vi "mono_camera.vi"(8 "error in":errorcluster, 11 "tcp_in":refnum<k5>) -> (0 "error out":errorcluster, 2 "camera_out":picture, 3 "tcp_out":refnum<k5>)   [LabVIEW 2018]
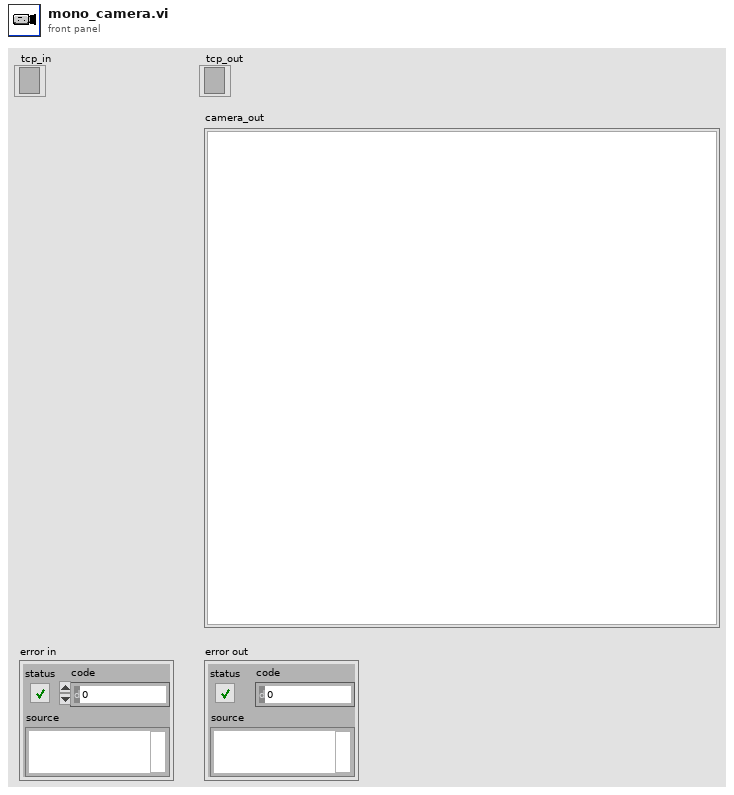
[diagram p1: front panel]
types:
  T1 = typedef "imagedata.ctl" = cluster{"image type":i32, "image depth":i32, "image":u8[], "mask":u8[], "colors":u32[], "Rectangle":cluster{"left":i16, "top":i16, "right":i16, "bottom":i16}}
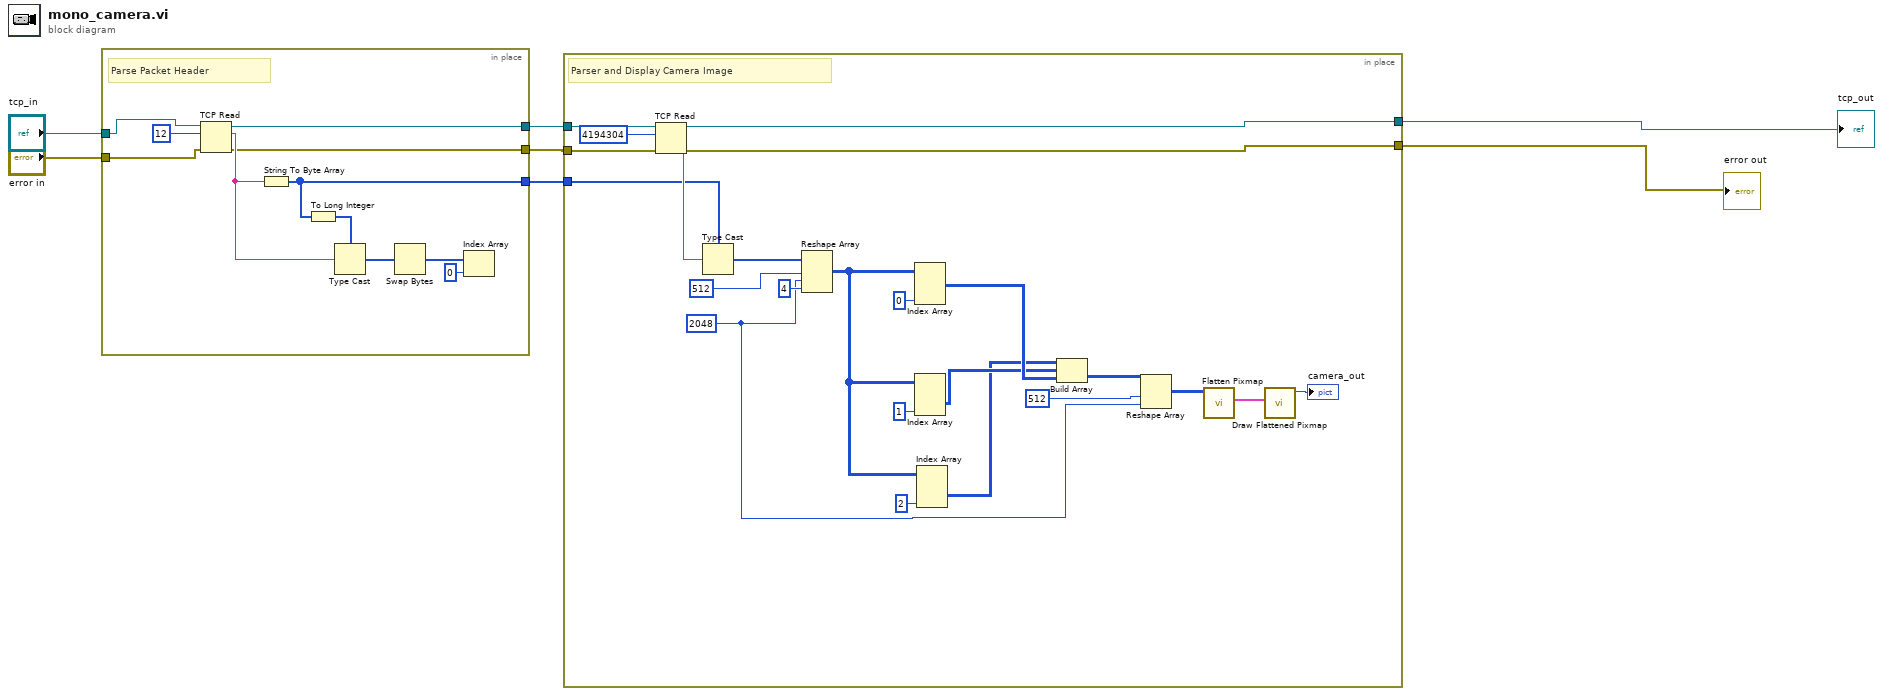
[diagram p0: block diagram]
diagram:
  n1 = in-place "Parse Header" {
    in-place-border: [w15] -> w1
    in-place-border: [w14] -> w2
    in-place-border: [w12] -> w3
    in-place-border: "error in" -> [w11]
    in-place-border: "tcp_in" -> [w10]
    # "Parse Packet Header"
    n2 = TCP Read(connection ID=w10, bytes to read=12, error in (no error)=w11) -> (connection ID out=w15:refnum<k5>, data out=w17:string, error out=w14:errorcluster)  [unwired: 2 in]
    n3 = String To Byte Array(string=w17) -> (unsigned byte array=w12:u8[])
    n4 = To Long Integer(number=w12) -> (32bit integer=w18:i32[])
    n5 = Type Cast(type=w18, x=w17) -> (*(type *) &x=w16:i32[])
    n6 = Swap Bytes(anything=w16) -> (byte swapped=w13:i32[])
    n7 = Index Array(array=w13, index=0) -> ()  [unwired: 1 out]
  }
  n8 = in-place {
    in-place-border: w1 -> [w41]
    in-place-border: w2 -> [w40]
    in-place-border: w3 -> [w38]
    in-place-border: [w32] -> w4
    in-place-border: [w31] -> w7
    w19 = 2048 ("dimension size")
    # "Parser and Display Camera Image"
    n9 = TCP Read(connection ID=w41, bytes to read=4194304, error in (no error)=w40) -> (connection ID out=w32:refnum<k5>, data out=w39:string, error out=w31:errorcluster)  [unwired: 2 in]
    n10 = Type Cast(type=w38, x=w39) -> (*(type *) &x=w22:u8[])
    n11 = Reshape Array(w22, 512 ("dimension size"), w19, 4 ("dimension size")) -> (w33:u8[][][])
    n12 = Index Array(array=w33, index (dim 2)=0 ("disabled index (col)")) -> (element=w25:u8[][])  [unwired: 2 in]
    n13 = Index Array(array=w33, index (dim 2)=1 ("index (col)")) -> (element=w24:u8[][])  [unwired: 2 in]
    n14 = Index Array(array=w33, index (dim 2)=2 ("index (col)")) -> (element=w23:u8[][])  [unwired: 2 in]
    n15 = Build Array(w23, w24, w25) -> (w29:u8[][][])
    n16 = Reshape Array(w29, 512 ("dimension size"), w19) -> (w26:u8[][])
    n17 = call <vilib>:"Flatten Pixmap.vi"("24-bit pixmap"=w26) -> ("image data"=w27:T1)  [unwired: 10 in]
    n18 = call <vilib>:"Draw Flattened Pixmap.vi"("image data"=w27) -> ("new picture"=→"camera_out":picture)  [unwired: 8 in]
  }
  "error out" <- w7
  "tcp_out" <- w4
